vi "Read Procedure Step Number.vi"(8 "error in":errorcluster, 11 "Console Log in":refnum<class "Console Log.lvclass">) -> (0 "error out":errorcluster, 2 "Step":i32, 3 "Console Log out":refnum<class "Console Log.lvclass">)   [LabVIEW 2011, in "Console Log.lvclass"]
uses:
  Console Log.lvclass
  Console Log.lvclass/Console Log.ctl
panel:
  out "text":string
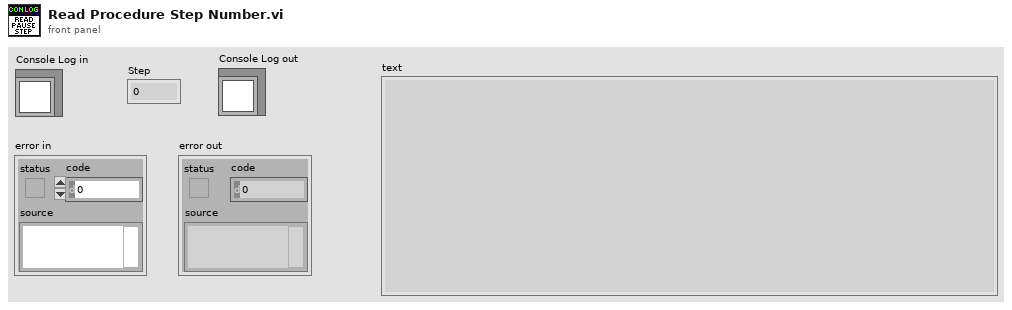
[diagram p1: front panel]
types:
  T1 = enum16{"open", "replace", "create", "open or create", "replace or create", "replace or create with confirmation"}
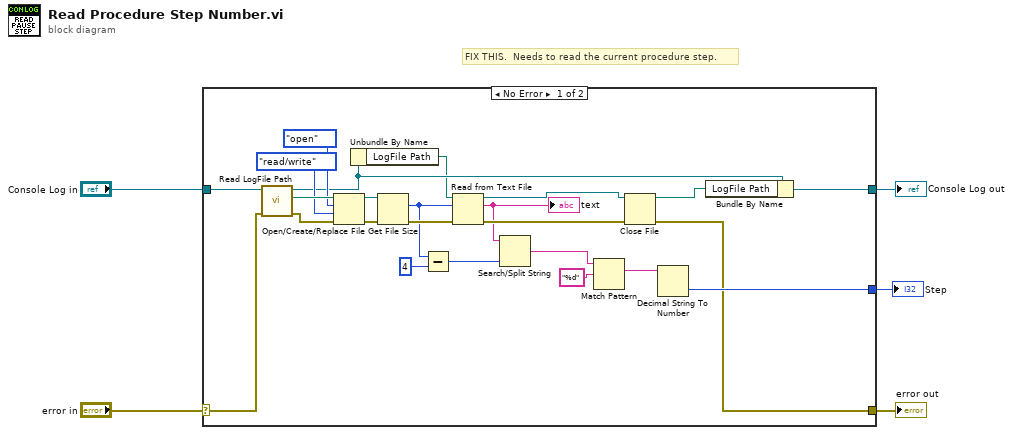
[diagram p0: block diagram]
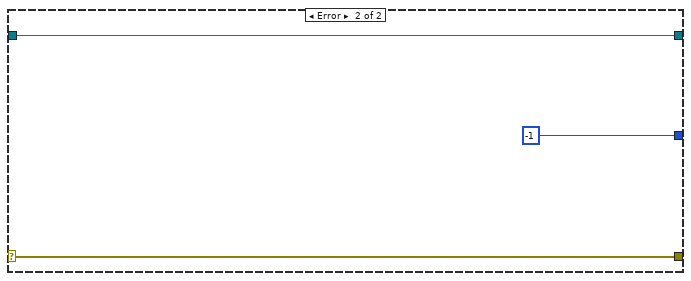
[diagram p2: hidden frame]
diagram:
  # "FIX THIS.  Needs to read the current procedure step."
  n1 = case shown="No Error" "error in" {
    selector: "error in" -> [w19 w32]
    tunnel: [w14 w32] -> w4
    tunnel: [w16 w31] -> w2
    tunnel: "Console Log in" -> [w23 w31]
    tunnel: [w20 -1] -> w1
    frame No Error {
      n2 = call "Read LogFile Path.vi"("error in (no error)"=w19, "Console Log in"=w23) -> ("error out"=w26:errorcluster, "LogFile Path"=w29:path, "Console Log out"=w13:refnum<class "Console Log.lvclass">)  [unwired: 7 in]
      n3 = Open/Create/Replace File(file path (use dialog)=w29, error in=w26, operation (0:open)=T1."open", access (0:read/write)=enum16{"read/write", "read-only", "write-only"}."read/write") -> (refnum out=w25:refnum<file>, error out=w24:errorcluster)  [unwired: 2 in, 1 out]
      n4 = Unbundle By Name(w13) -> ("LogFile Path"=w12:path)
      n5 = Get File Size(file=w25, error in=w24) -> (size (in bytes)=w9:i64, 0:w11:errorcluster)  [unwired: 1 out]
      n6 = Subtract(x=w9, y=i64 4) -> (x-y=w7:i64)
      n7 = Read from Text File(file (use dialog)=w12, count=w9, error in=w11) -> (refnum out=w18:refnum<file>, text=w10:string, error out=w17:errorcluster)  [unwired: 1 in, 1 out]
      "text" <- w10
      n8 = Search/Split String(string=w10, offset (0)=w7) -> (match + rest of string=w6:string)  [unwired: 1 in, 2 out]
      n9 = Match Pattern(string=w6, regular expression="%d") -> (match substring=w21:string)  [unwired: 1 in, 3 out]
      n10 = Close File(refnum=w18, error in=w17) -> (path=w15:path, error out=w14:errorcluster)
      n11 = Decimal String To Number(string=w21) -> (number=w20:i32)  [unwired: 2 in, 1 out]
      n12 = Bundle By Name(cluster=w13, "LogFile Path"=w15) -> (w16:refnum<class "Console Log.lvclass">)
    }
    frame Error {
    }
  }
  "error out" <- w4
  "Console Log out" <- w2
  "Step" <- w1
